vi "Read Vertical Scroll.vi"(8 "error in (no error)":errorcluster, 11 "Pane in":refnum<class "Pane.lvclass">) -> (0 "error out":errorcluster, 2 "Horizontal Scroll":T1 caption="Vertical Scroll", 3 "Pane out":refnum<class "Pane.lvclass">)   [LabVIEW 2017, in "Pane.lvclass"]
uses:
  Pane.lvclass
  Typedefs/Scrollbar Visibility--Enum.ctl
  Pane.lvclass/Pane.ctl
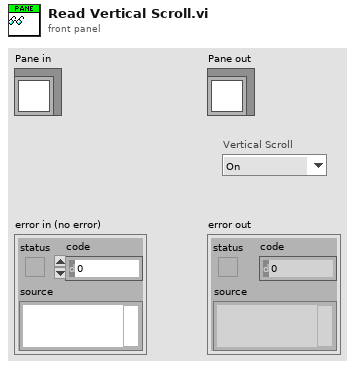
[diagram p1: front panel]
types:
  T1 = typedef "Scrollbar Visibility--Enum.ctl" = enum16{"On", "Off", "Off (Runtime)"}
  T2 = enum16{"Always On", "Always Off", "Off While Running"}
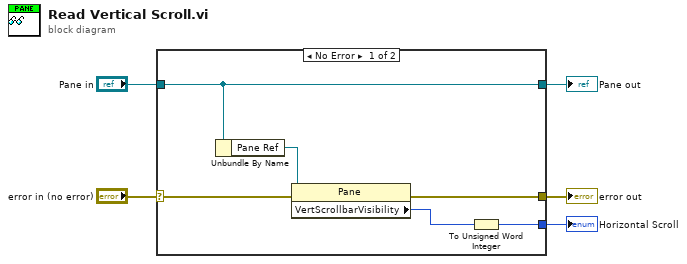
[diagram p0: block diagram]
diagram:
  n1 = case shown="No Error" "error in (no error)" {
    selector: "error in (no error)" -> [w11 w12]
    tunnel: [w9 w12] -> w4
    tunnel: [w10 w13] -> w2
    tunnel: "Pane in" -> [w10 w13]
    tunnel: [w6 _] -> w1
    frame No Error {
      n2 = Unbundle By Name(w10) -> ("Pane Ref"=w8:refnum<vi>)
      n3 = property class="Pane"(reference=w8, error in=w11) -> (error out=w9:errorcluster, "VertScrollbarVisibility"=w7:T2)  [unwired: 1 out]
      n4 = To Unsigned Word Integer(number=w7) -> (unsigned 16bit integer=w6:u16)
    }
    frame Error {
    }
  }
  "error out" <- w4
  "Pane out" <- w2
  "Horizontal Scroll" <- w1
